vi "hashead.vi"(11 "port":refnum<visa-resource-name>) -> (3 "has head":bool)   [LabVIEW 2012]
uses:
  <vilib>/Instr/_visa.llb/VISA Configure Serial Port (Instr).vi
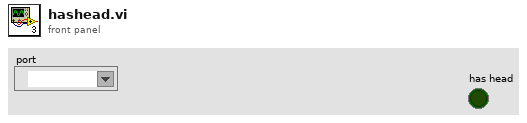
[diagram p1: front panel]
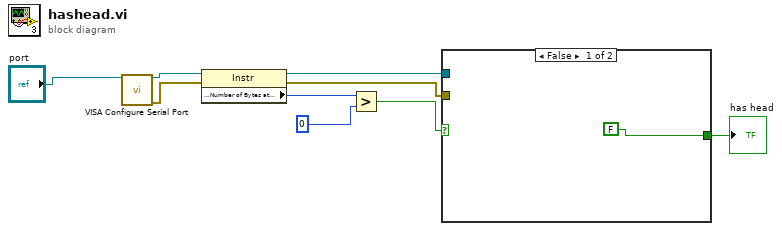
[diagram p0: block diagram]
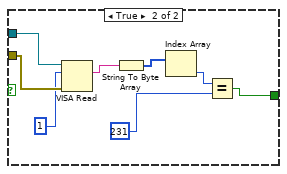
[diagram p2: hidden frame]
diagram:
  n1 = call-poly "VISA Configure Serial Port"("VISA resource name"="port") -> ("VISA resource name out"=w8:refnum<visa-resource-name>, "error out"=w7:errorcluster)  [unwired: 13 in]
  n2 = property class="Instr"(reference=w8, error in=w7) -> (reference out=w3:refnum<visa-resource-name>, error out=w2:errorcluster, "Serial Settings:Number of Bytes at Serial Port"=w5:u32)
  n3 = Greater?(x=w5, y=0) -> (0:w4:bool)
  n4 = case shown="False" w4 {
    tunnel: w3 -> [_ w18]
    tunnel: w2 -> [_ w17]
    tunnel: [FALSE w11] -> w1
    frame False {
    }
    frame True {
      n5 = VISA Read(VISA resource name=w18, byte count=1, error in (no error)=w17) -> (read buffer=w14:string)  [unwired: 3 out]
      n6 = String To Byte Array(string=w14) -> (unsigned byte array=w13:u8[])
      n7 = Index Array(array=w13) -> (element=w12:u8)  [unwired: 1 in]
      n8 = Equal?(x=w12, y=u8 231) -> (x = y?=w11:bool)
    }
  }
  "has head" <- w1
